vi "when_pressed.vi"(11 "Input":bool) -> (3 "Output":bool)   [LabVIEW 2020]
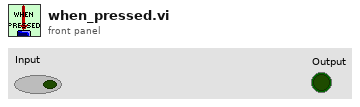
[diagram p1: front panel]
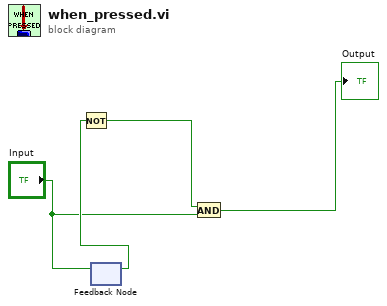
[diagram p0: block diagram]
diagram:
  n1 = feedback #1() -> (w3:bool)  [unwired: 1 in]
  n2 = Not(x=w3) -> (.not. x?=w2:bool)
  n3 = feedback-in #1("Input") -> ()
  n4 = And(x=w2, y="Input") -> (x .and. y?=→"Output":bool)
